vi "storeControlXML.vi"(2 "XMLoption":T1, 3 "Error In":errorcluster, 4 "CallerVIref":refnum<vi>, 5 "Control References":refnum<vi>[](array[refnum])) -> (0 "Error Out":errorcluster)   [LabVIEW 2012]
uses:
  controls/XmlOption.ctl
  <vilib>/Utility/xml.llb/Write to XML File(array).vi
  <vilib>/Utility/xml.llb/Read From XML File(array).vi
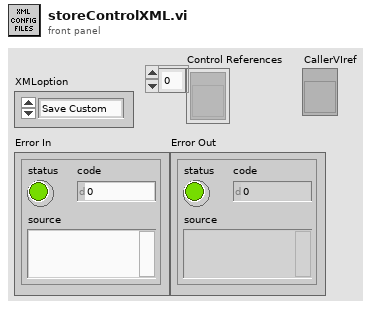
[diagram p1: front panel]
types:
  T1 = typedef "XmlOption.ctl" = enum16{"Save Custom", "Load Custom", "Save Default", "Load Default"}
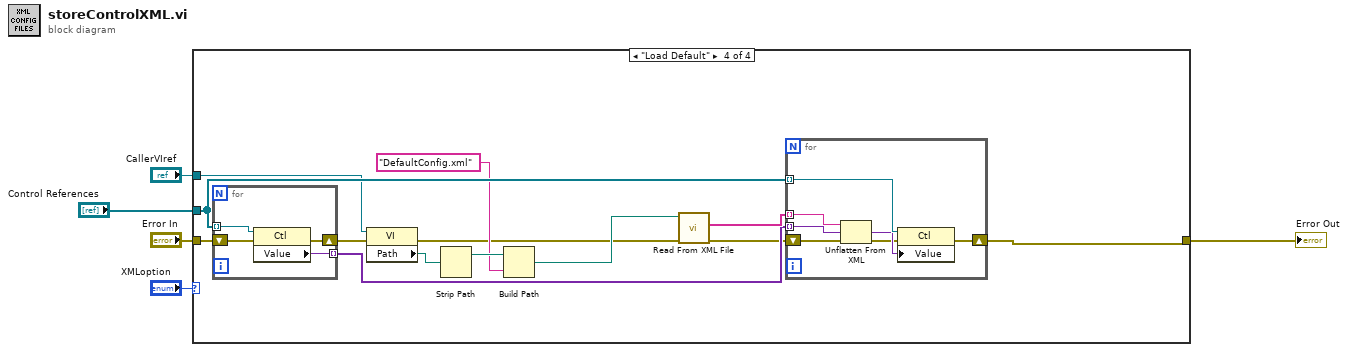
[diagram p0: block diagram]
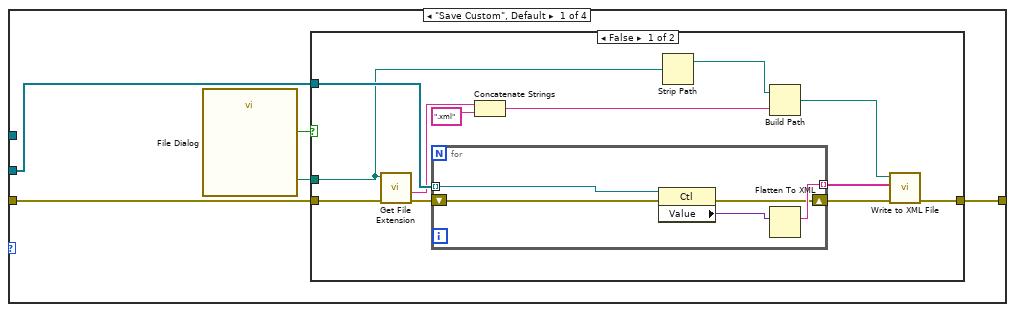
[diagram p2: hidden frame]
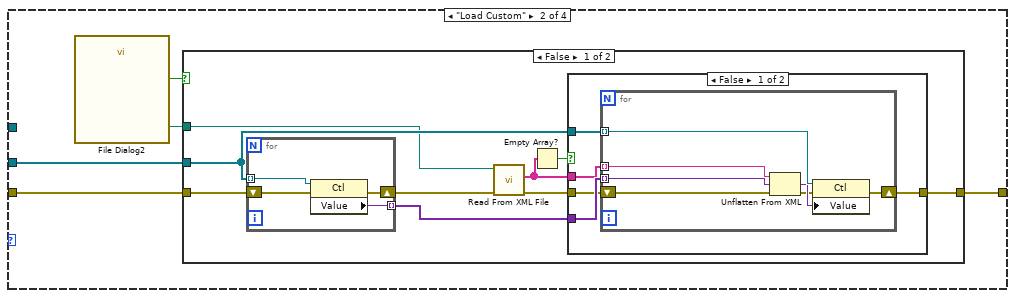
[diagram p4: hidden frame]
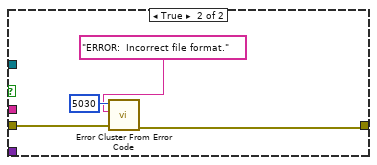
[diagram p5: hidden frame]
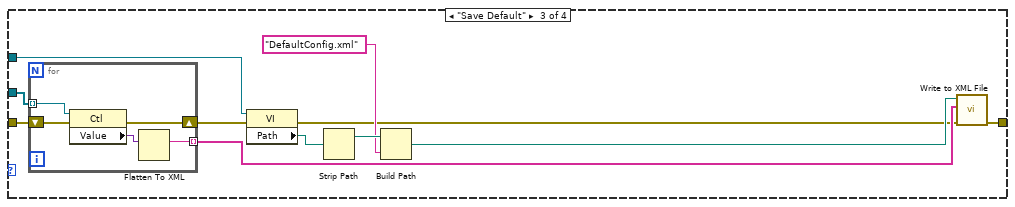
[diagram p7: hidden frame]
diagram:
  n1 = case shown="\"Load Default\"" "XMLoption" {
    tunnel: "Control References" -> [w10 w32 w74 w90]
    tunnel: "CallerVIref" -> [_ _ w69 w84]
    tunnel: "Error In" -> [w9 w31 w67 w86]
    tunnel: [w6 w33 w64 w80] -> w1
    frame "Save Custom", Default {
      n2 = call "File Dialog"() -> ("selected path"=w7:path, "cancelled"=w8:bool)  [unwired: 12 in, 2 out]
      n3 = case shown="False" w8 {
        tunnel: w10 -> [w21 _]
        tunnel: w9 -> [w20 w28]
        tunnel: w7 -> [w15 _]
        tunnel: [w11 w28] -> w6
        frame False {
          n4 = call <vilib>:"Get File Extension.vi"("error in (no error)"=w20, "file"=w15) -> ("error out"=w19:errorcluster, "filename without extension"=w18:string)  [unwired: 6 in, 2 out]
          n5 = for {
            tunnel: w21 -> [w27] mode=indexing
            tunnel: [w26] -> w22 mode=indexing
            shift-right: [w23] -> w16
            shift-left: w19 -> [w24]
            n6 = property class="Ctl"(reference=w27, error in=w24) -> (error out=w23:errorcluster, "Value"=w25:variant)  [unwired: 1 out]
            n7 = Flatten To XML(anything=w25) -> (xml string=w26:string)
          }
          n8 = Concatenate Strings(w18, ".xml" ("string")) -> (w13:string)
          n9 = Strip Path(path=w15) -> (stripped path=w14:path)  [unwired: 1 out]
          n10 = Build Path(base path=w14, name or relative path=w13) -> (appended path=w12:path)
          n11 = call-poly <vilib>:"Write to XML File.vi"("error in (no error)"=w16, "XML Input"=w22, "XML File Path"=w12) -> ("error out"=w11:errorcluster)  [unwired: 6 in, 2 out]
        }
        frame True {
        }
      }
    }
    frame "Load Custom" {
      n12 = call "File Dialog2"() -> ("selected path"=w29:path, "cancelled"=w30:bool)  [unwired: 12 in, 2 out]
      n13 = case shown="False" w30 {
        tunnel: [w39 w63] -> w33
        tunnel: w32 -> [w38 _]
        tunnel: w31 -> [w37 w63]
        tunnel: w29 -> [w36 _]
        frame False {
          n14 = for {
            tunnel: w38 -> [w62] mode=indexing
            shift-right: [w60] -> w42
            shift-left: w37 -> [w61]
            tunnel: [w59] -> w41 mode=indexing
            n15 = property class="Ctl"(reference=w62, error in=w61) -> (error out=w60:errorcluster, "Value"=w59:variant)  [unwired: 1 out]
          }
          n16 = call-poly <vilib>:"Read From XML File.vi"("error in (no error)"=w42, "XML File Path"=w36) -> ("error out"=w40:errorcluster, "XML Elements"=w35:string[])  [unwired: 7 in, 1 out]
          n17 = Empty Array?(array=w35) -> (empty?=w34:bool)
          n18 = case shown="False" w34 {
            tunnel: w41 -> [w47 _]
            tunnel: w40 -> [w46 w58]
            tunnel: [w45 w57] -> w39
            tunnel: w38 -> [w44 _]
            tunnel: w35 -> [w43 _]
            frame False {
              n19 = for {
                tunnel: w44 -> [w54] mode=indexing
                tunnel: w47 -> [w52] mode=indexing
                tunnel: w43 -> [w53] mode=indexing
                shift-right: [w48] -> w45
                shift-left: w46 -> [w50]
                n20 = Unflatten From XML(xml string=w53, type=w52, error in (no error)=w50) -> (value=w51:variant, error out=w49:errorcluster)
                n21 = property class="Ctl"(reference=w54, error in=w49, "Value"=w51) -> (error out=w48:errorcluster)  [unwired: 1 out]
              }
            }
            frame True {
              n22 = call <vilib>:"Error Cluster From Error Code.vi"("error in (no error)"=w58, "error message (\"\")"="ERROR:  Incorrect file format.", "error code (0)"=5030) -> ("error out"=w57:errorcluster)  [unwired: 6 in]
            }
          }
        }
        frame True {
        }
      }
    }
    frame "Save Default" {
      n23 = for {
        tunnel: w74 -> [w79] mode=indexing
        tunnel: [w78] -> w73 mode=indexing
        shift-right: [w75] -> w66
        shift-left: w67 -> [w76]
        n24 = property class="Ctl"(reference=w79, error in=w76) -> (error out=w75:errorcluster, "Value"=w77:variant)  [unwired: 1 out]
        n25 = Flatten To XML(anything=w77) -> (xml string=w78:string)
      }
      n26 = property class="VI"(reference=w69, error in=w66) -> (error out=w65:errorcluster, "Path"=w71:path)  [unwired: 1 out]
      n27 = Strip Path(path=w71) -> (stripped path=w72:path)  [unwired: 1 out]
      n28 = Build Path(base path=w72, name or relative path="DefaultConfig.xml") -> (appended path=w68:path)
      n29 = call-poly <vilib>:"Write to XML File.vi"("error in (no error)"=w65, "XML Input"=w73, "XML File Path"=w68) -> ("error out"=w64:errorcluster)  [unwired: 6 in, 2 out]
    }
    frame "Load Default" {
      n30 = for {
        tunnel: w90 -> [w96] mode=indexing
        shift-right: [w94] -> w85
        shift-left: w86 -> [w95]
        tunnel: [w93] -> w91 mode=indexing
        n31 = property class="Ctl"(reference=w96, error in=w95) -> (error out=w94:errorcluster, "Value"=w93:variant)  [unwired: 1 out]
      }
      n32 = property class="VI"(reference=w84, error in=w85) -> (error out=w82:errorcluster, "Path"=w88:path)  [unwired: 1 out]
      n33 = Strip Path(path=w88) -> (stripped path=w89:path)  [unwired: 1 out]
      n34 = Build Path(base path=w89, name or relative path="DefaultConfig.xml") -> (appended path=w83:path)
      n35 = call-poly <vilib>:"Read From XML File.vi"("error in (no error)"=w82, "XML File Path"=w83) -> ("error out"=w81:errorcluster, "XML Elements"=w92:string[])  [unwired: 7 in, 1 out]
      n36 = for {
        tunnel: w90 -> [w103] mode=indexing
        tunnel: w91 -> [w101] mode=indexing
        tunnel: w92 -> [w102] mode=indexing
        shift-right: [w97] -> w80
        shift-left: w81 -> [w99]
        n37 = Unflatten From XML(xml string=w102, type=w101, error in (no error)=w99) -> (value=w100:variant, error out=w98:errorcluster)
        n38 = property class="Ctl"(reference=w103, error in=w98, "Value"=w100) -> (error out=w97:errorcluster)  [unwired: 1 out]
      }
    }
  }
  "Error Out" <- w1
